vi "LED Execute.vi"() -> ()   [LabVIEW 2017]
uses:
  <vilib>/Rock Robotics/WPI/ThirdParty/Phoenix-LabVIEW/CANifier/CTRE_CANifier_LEDChannel.ctl
  LED Control Type.ctl
  <vilib>/Rock Robotics/WPI/DriverStation/WPI_DriverStationRobotMode2.ctl
  LED Notifier.ctl
  LED Globals.vi
  Utility VIs/Refnum Names.vi
  Robot Global Data.vi
panel:
  out "error out":errorcluster
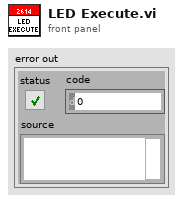
[diagram p1: front panel]
types:
  T1 = typedef "CTRE_CANifier_DeviceRef.ctl" = cluster{"DeviceStatus":errorcluster, "Device Number":u8, "Handle":u64, "UsageFrame":u32, "Library Path":path}
  T2 = typedef "LED Control Type.ctl" = enum16{"Off", "Waiting On Field", "Connected ", "Cube In Intake", "Climbing", "Auto Cube Capture", "Ready for Cube Floor", "Ready for Cube Portal"}
  T3 = typedef "CTRE_CANifier_LEDChannel.ctl" = enum32{"LEDChannelA", "LEDChannelB", "LEDChannelC"}
  T4 = typedef "LED Notifier.ctl" = cluster{"LED Control Type":T2, "Climbing":bool, "Auto Tracking":bool, "Ready for Cube Floor":bool, "Ready for Cube Portal":bool}
  T5 = typedef "WPI_DriverStationRobotMode2.ctl" = enum16{"Autonomous Disabled", "Autonomous Enabled", "Teleop Disabled", "Teleop Enabled", "Disconnected", "Finish", "Test Disabled", "Test Enabled", "Emergency Stopped"}
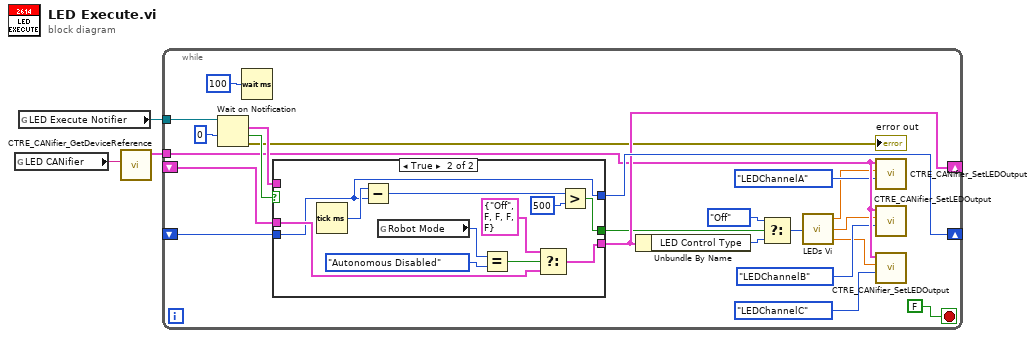
[diagram p0: block diagram]
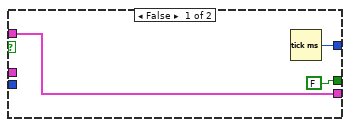
[diagram p2: hidden frame]
diagram:
  n1 = global read "Refnum Names.vi" "LED CANifier"() -> (w1:string)
  n2 = global read "LED Globals.vi" "LED Execute Notifier"() -> (w3:refnum<notifier>)
  n3 = call <vilib>:"CTRE_CANifier_GetDeviceReference.vi"("refnum name"=w1) -> ("CANifierDevRef"=w2:T1)  [unwired: 9 in, 1 out]
  n4 = while {
    tunnel: w3 -> [w23]
    shift-right: [w16] -> _
    shift-left: _ -> [w20]
    shift-right: [w18] -> _
    shift-left: _ -> [w17]
    tunnel: w2 -> [w13]
    stop <- FALSE stop-if-true
    n5 = Wait on Notification(notifier=w23, timeout in ms (-1)=0) -> (notification=w19:T4, timed out?=w21:bool, error out=→"error out":errorcluster)  [unwired: 2 in, 1 out]
    n6 = Wait (ms)(milliseconds to wait=u32 100) -> ()  [unwired: 1 out]
    n7 = case shown="True" w21 {
      tunnel: w20 -> [_ w38]
      tunnel: [w28 w37] -> w16
      tunnel: w19 -> [w28 _]
      tunnel: [w27 w30] -> w18
      tunnel: w17 -> [_ w30]
      tunnel: [FALSE w33] -> w14
      frame False {
        n8 = Tick Count (ms)() -> (millisecond timer value=w27:u32)
      }
      frame True {
        n9 = Tick Count (ms)() -> (millisecond timer value=w36:u32)
        n10 = Subtract(x=w36, y=w30) -> (x-y=w35:u32)
        n11 = global read "Robot Global Data.vi" "Robot Mode"() -> (w32:T5)
        n12 = Equal?(x=w32, y=WPI_DriverStationRobotMode2."Autonomous Disabled") -> (x = y?=w39:bool)
        n13 = Select(t=T4 {"LED Control Type"=enum."Off", "Climbing"=FALSE, "Auto Tracking"=FALSE, "Ready for Cube Floor"=FALSE, "Ready for Cube Portal"=FALSE} ("LED Notifier"), s=w39, f=w38) -> (s? t:f=w37:T4)
        n14 = Greater?(x=w35, y=u32 500) -> (0:w33:bool)
      }
    }
    n15 = Unbundle By Name(w16) -> ("LED Control Type"=w15:T2)
    n16 = Select(t=LED_Control_Type."Off", s=w14, f=w15) -> (s? t:f=w5:T2)
    n17 = call "LEDs Vi.vi"("LED Control Type"=w5) -> ("G"=w6:dbl, "B"=w7:dbl, "R"=w8:dbl)  [unwired: 2 in]
    n18 = call <vilib>:"CTRE_CANifier_SetLEDOutput.vi"("LEDChannel"=CTRE_CANifier_LEDChannel."LEDChannelA", "Percent Output"=w8, "CANifierDevRef"=w13) -> ()  [unwired: 7 in, 2 out]
    n19 = call <vilib>:"CTRE_CANifier_SetLEDOutput.vi"("LEDChannel"=CTRE_CANifier_LEDChannel."LEDChannelB", "Percent Output"=w7, "CANifierDevRef"=w13) -> ()  [unwired: 7 in, 2 out]
    n20 = call <vilib>:"CTRE_CANifier_SetLEDOutput.vi"("LEDChannel"=CTRE_CANifier_LEDChannel."LEDChannelC", "Percent Output"=w6, "CANifierDevRef"=w13) -> ()  [unwired: 7 in, 2 out]
  }
